vi "sound.vi"() -> ()   [LabVIEW 2013]
uses:
  <vilib>/sound2/lvsound2.llb/Sampling Mode.ctl
  <vilib>/sound2/lvsound2.llb/Sound Data Format.ctl
  <vilib>/sound2/lvsound2.llb/Sound Output Set Volume (Single).vi
  <vilib>/sound2/lvsound2.llb/Sound Output Write (DBL Single).vi
panel:
  in  "Knob":dbl(knob) scale=0.0..30000.0
  in  "Device ID":u32
  in  "Stop":bool
  out "Frequency":dbl=500.0
  out "Generated Sound":waveform(dbl)(graph)
  in  "Volume":dbl(slide)=50.0 scale=0.0..100.0
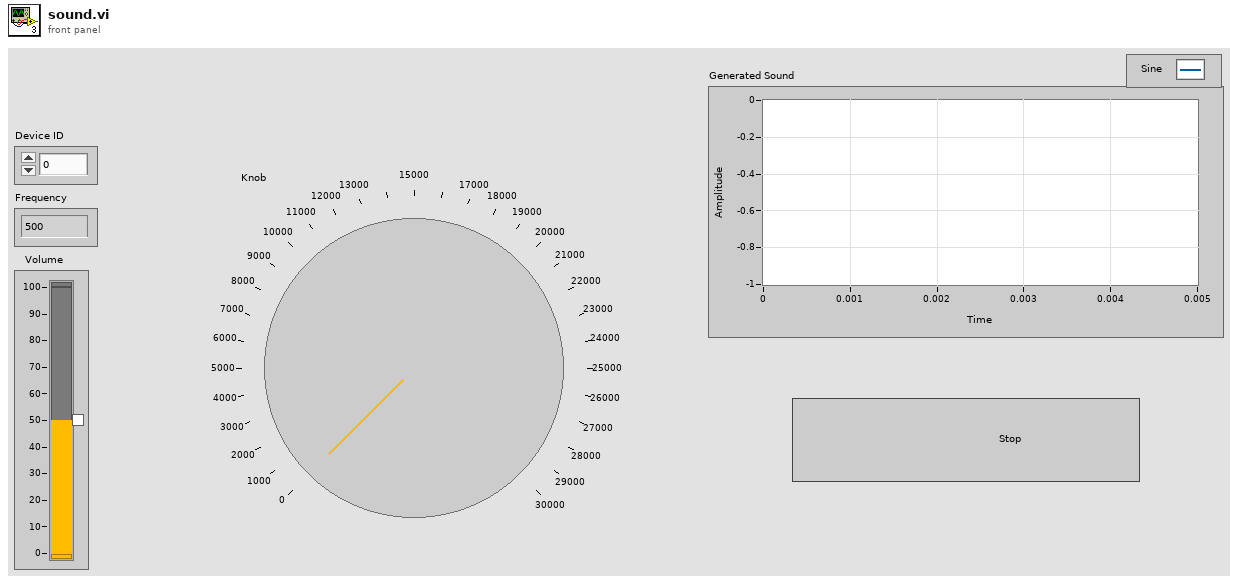
[diagram p1: front panel]
types:
  T1 = typedef "Sound Data Format.ctl" = cluster{"sample rate (S/s)":dbl, "number of channels":i32, "bits per sample":i32}
  T2 = typedef "Sampling Mode.ctl" = i32
  T3 = typedef "Sound Output Task ID.ctl" = u32
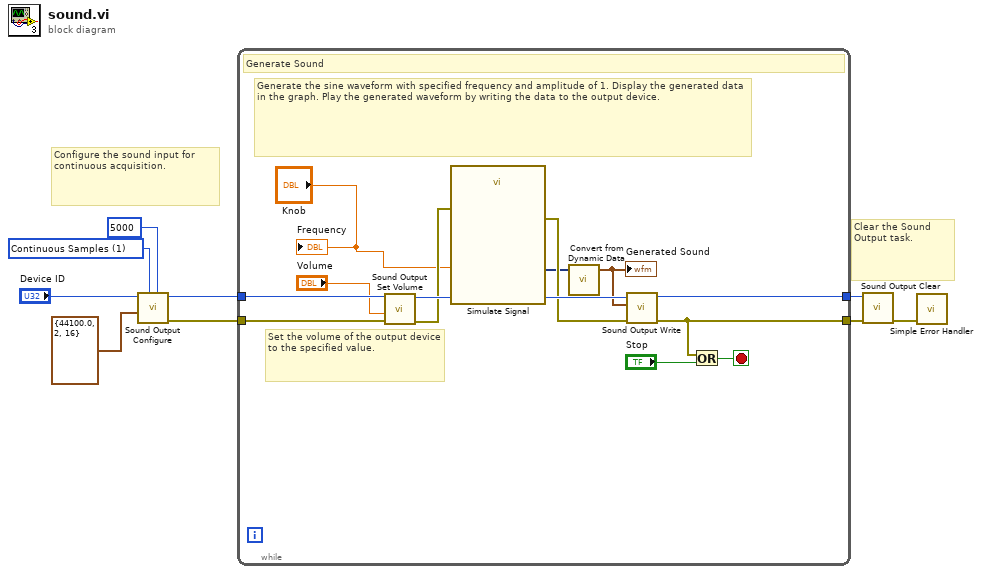
[diagram p0: block diagram]
diagram:
  w4 = T2 1 items=["Finite Samples", "Continuous Samples"] ("sample mode")
  # "Configure the sound input for continuous acquisition."
  # "Clear the Sound Output task."
  n1 = call <vilib>:"Sound Output Configure.vi"("number of samples/ch"=5000 ("Number of Samples/ch"), "sample mode"=w4, "sound format"=T1 {"sample rate (S/s)"=44100.0, "number of channels"=2, "bits per sample"=16} ("Sound Format"), "device ID"="Device ID") -> ("error out"=w9:errorcluster, "task ID"=w8:T3)  [unwired: 6 in]
  n2 = while {
    tunnel: w8 -> [w17]
    tunnel: [w22] -> w6
    tunnel: w9 -> [w19]
    tunnel: [w15] -> w7
    stop <- w20 stop-if-true
    # "Set the volume of the output device to the specified value."
    # "Generate the sine waveform with specified frequency and amplitude of 1. Display the generated data in the graph. Play the generated waveform by writing the data to the output device."
    # "Generate Sound"
    n3 = call-poly <vilib>:"Sound Output Set Volume.vi"("error in (no error)"=w19, "volume"="Volume", "task ID"=w17) -> ("error out"=w13:errorcluster, "task ID out"=w18:T3)  [unwired: 7 in]
    n4 = call "Simulate Signal"("Frequency"="Knob", "error in (no error)"=w13) -> ("Sine"=w11:dynamicdata, "error out"=w12:errorcluster)  [unwired: 12 in]
    n5 = call "Convert from Dynamic Data"("Dynamic Data Type"=w11) -> ("Waveform"=w14:waveform(dbl))  [unwired: 3 in]
    "Generated Sound" <- w14
    n6 = call-poly <vilib>:"Sound Output Write.vi"("error in (no error)"=w12, "data"=w14, "task ID"=w18) -> ("error out"=w15:errorcluster, "task ID out"=w22:T3)  [unwired: 7 in]
    n7 = Or(x=w15, y="Stop") -> (x .or. y?=w20:bool)
    "Frequency" <- "Knob"
  }
  n8 = call <vilib>:"Sound Output Clear.vi"("error in (no error)"=w7, "task ID"=w6) -> ("error out"=w2:errorcluster)  [unwired: 9 in]
  n9 = call <vilib>:"Simple Error Handler.vi"("error in (no error)"=w2) -> ()  [unwired: 4 in, 5 out]
